vi "Conveyor and Shoot Logging Values.vi"() -> ()   [LabVIEW 2016]
panel:
  out "Shooter Slave Current":dbl
  out "Shooter Master Current":dbl
  out "Flywheel Actual Velocity":dbl
  out "Flywheel Commanded Velocity":dbl
  out "Conveyor Speed":dbl
  out "Manual Reverse Conveyor":bool
  out "Run Feed System":bool
  out "Toggle Shooter":bool
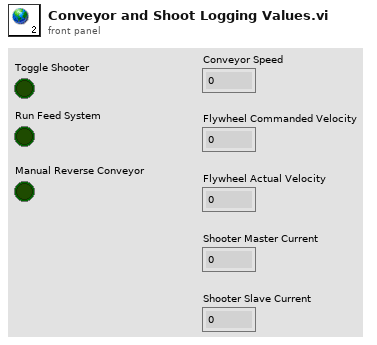
[diagram p1: front panel]
diagram:
